vi "GOO.vi"() -> ()   [LabVIEW 2010]
panel:
  in  "Начать тестирование":bool
  in  "БУС":bool
  in  "БВ":bool
  in  "Виртуальный объект управления":bool
  in  "Алгоритм управления":bool
  in  "Ручное/Автоматическое управление":bool
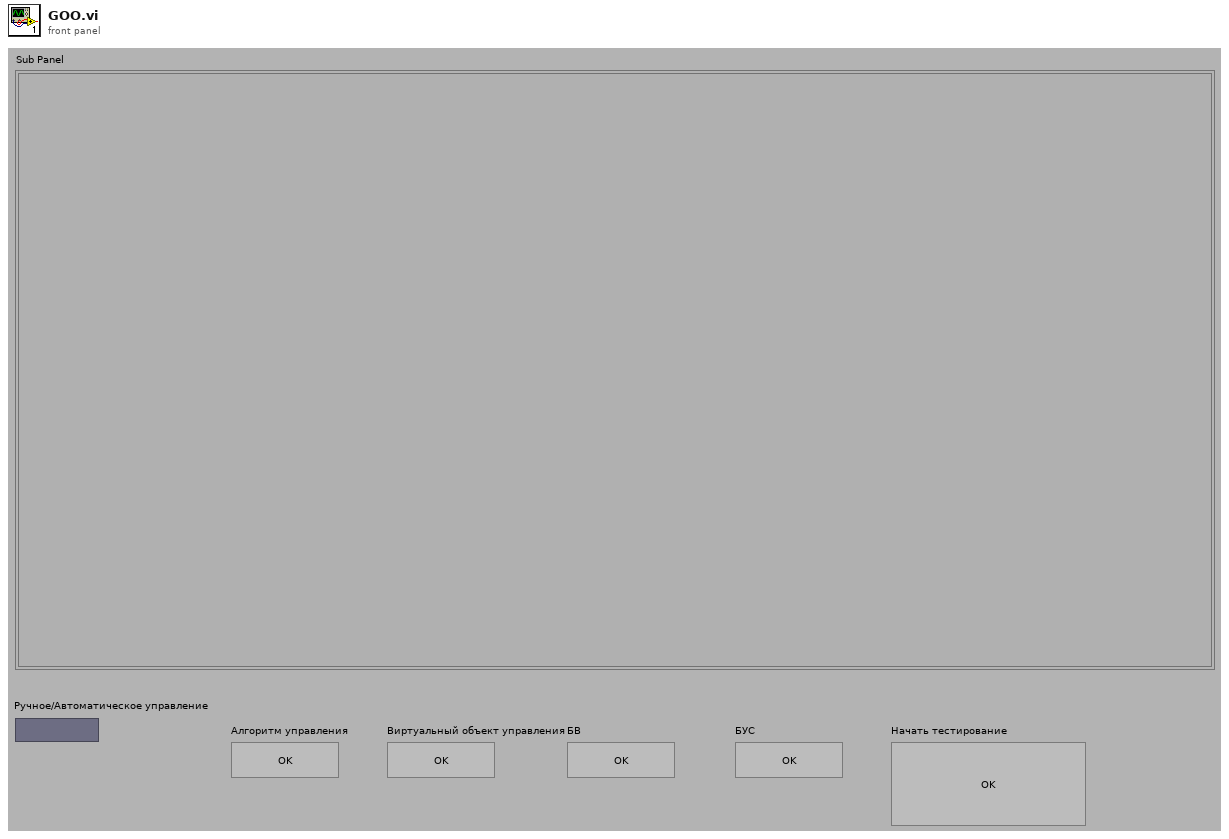
[diagram p1: front panel]
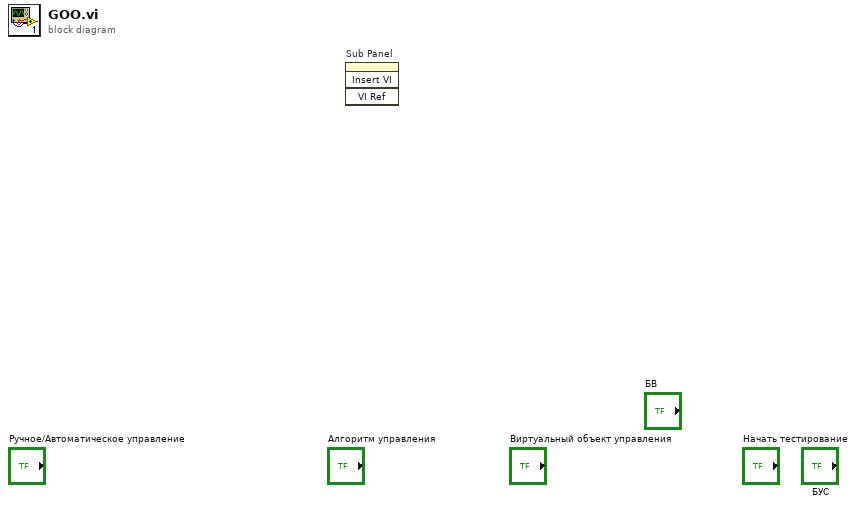
[diagram p0: block diagram]
diagram:
  n1 = invoke on="Sub Panel" class="SubPanel" method="Insert VI"() -> ()  [unwired: 4 in, 4 out]
